vi "Set UDP Destination Port.vi"(0 "Refnum in":refnum<k20>, 5 "ethernet port":i32, 7 "UDP Destination Port":u16, 11 "error in (no error)":errorcluster) -> (4 "Refnum out":refnum<k20>, 15 "error out":errorcluster)   [LabVIEW 2020, in "My Network Host v1.lvlib"]
uses:
  My Network Host v1.lvlib
  <vilib>/Utility/error.llb/Error Cluster From Error Code.vi
  <vilib>/rvi/errors/niLvFpgaAdjustHostInterfaceError.vi
  <vilib>/rvi/interface/nirviReadWriteControl/nirviReadWriteControl.xnode
  NiFpgaLv.dll
  <vilib>/rvi/interface/Simulation/niFpgaSimulationCallBeginRW.vi
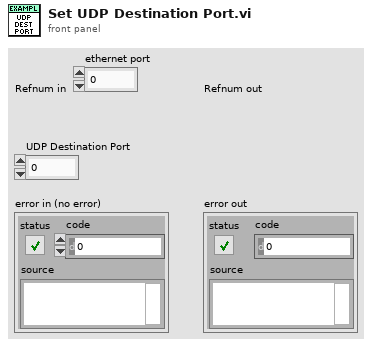
[diagram p1: front panel]
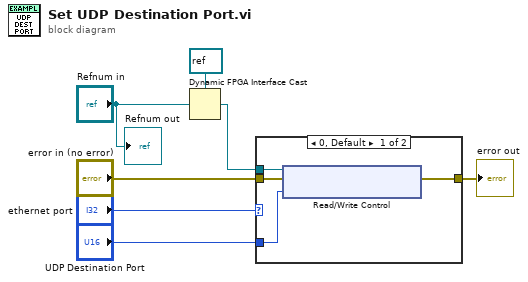
[diagram p0: block diagram]
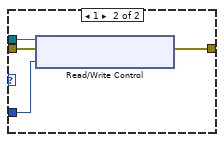
[diagram p2: hidden frame]
diagram:
  n1 = Dynamic FPGA Interface Cast(Session In=refnum<k20> refnum ("FPGA VI Reference In"), Type="Refnum in") -> (Session Out=w4:refnum<k20>)
  n2 = case shown="0, Default" "ethernet port" {
    tunnel: [w11 w15] -> w7
    tunnel: "error in (no error)" -> [w10 w14]
    tunnel: "UDP Destination Port" -> [w9 w13]
    tunnel: w4 -> [w8 w12]
    frame 0, Default {
      n3 = xnode "Read/Write Control"("FPGA VI Reference In"=w8, "error in"=w10, "UDP Destination Port 0"=w9) -> ("error out"=w11:errorcluster)  [unwired: 1 out]
    }
    frame 1 {
      n4 = xnode "Read/Write Control"("FPGA VI Reference In"=w12, "error in"=w14, "UDP Destination Port 1"=w13) -> ("error out"=w15:errorcluster)  [unwired: 1 out]
    }
  }
  "error out" <- w7
  "Refnum out" <- "Refnum in"
